vi "CRYSet Hardware Editor Front Panel.vi"(11 "Vi Ref":refnum<vi>) -> ()   [LabVIEW 2013]
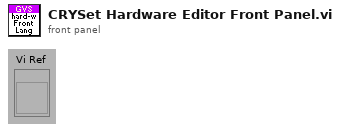
[diagram p1: front panel]
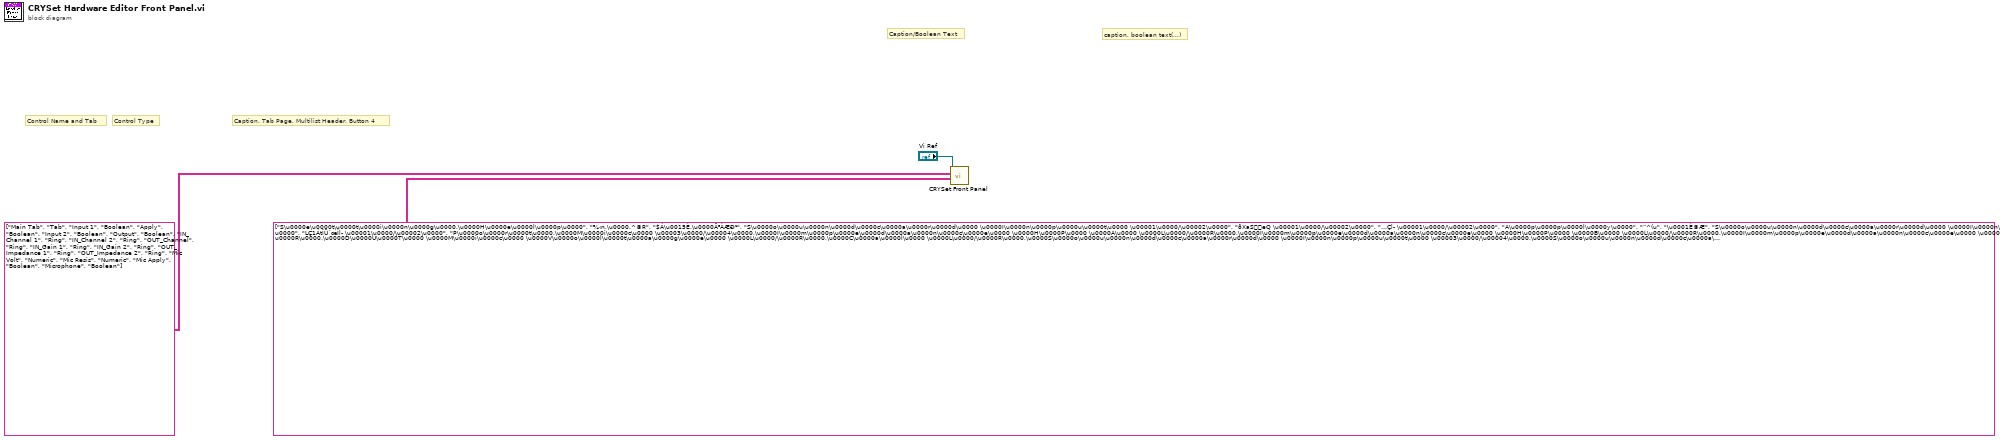
[diagram p0: block diagram]
diagram:
  # "Caption, Tab Page, Multilist Header, Button 4"
  # "Control Type"
  # "Control Name and Tab"
  # "caption, boolean text(,,,)"
  # "Caption/Boolean Text"
  n1 = call "CRYSet Front Panel.vi"("Caption(Boolean Text)"=string[][] [["S\u0000e\u0000t\u0000t\u0000i\u0000n\u0000g\u0000,\u0000H\u0000e\u0000l\u0000p\u0000", "¾‹n,\u0000.^©R", "$Á\u0015È,\u0000Ä³ÀÆÐ¹"], ["S\u0000o\u0000u\u0000n\u0000d\u0000c\u0000a\u0000r\u0000d\u0000 \u0000I\u0000n\u0000p\u0000u\u0000t\u0000 \u00001\u0000/\u00002\u0000", "ðXaSeQ \u00001\u0000/\u00002\u0000", "…Çl­ \u00001\u0000/\u00002\u0000"], ["A\u0000p\u0000p\u0000l\u0000y\u0000", "”^(u", "\u0001È©Æ"], ["S\u0000o\u0000u\u0000n\u0000d\u0000c\u0000a\u0000r\u0000d\u0000 \u0000I\u0000n\u0000p\u0000u\u0000t\u0000 \u00003\u0000/\u00004\u0000", "ðXaSeQ \u00003\u0000/\u00004\u0000", "LÇ1ÁtÎÜ´…Çl­ \u00001\u0000/\u00002\u0000"], ["S\u0000o\u0000u\u0000n\u0000d\u0000c\u0000a\u0000r\u0000d\u0000 \u0000O\u0000u\u0000t\u0000p\u0000u\u0000t\u0000 \u00001\u0000/\u00002\u0000", "ðXaSúQ \u00001\u0000/\u00002\u0000", "LÇ1ÁtÎÜ´œÍl­ \u00001\u0000/\u00002\u0000"], ["P\u0000o\u0000r\u0000t\u0000,\u0000M\u0000i\u0000c\u0000 \u00003\u0000/\u00004\u0000,\u0000I\u0000m\u0000p\u0000e\u0000d\u0000a\u0000n\u0000c\u0000e\u0000 \u0000H\u0000P\u0000 \u0000A\u0000 \u0000L\u0000/\u0000R\u0000,\u0000I\u0000m\u0000p\u0000e\u0000d\u0000a\u0000n\u0000c\u0000e\u0000 \u0000H\u0000P\u0000 \u0000B\u0000 \u0000L\u0000/\u0000R\u0000,\u0000I\u0000m\u0000p\u0000e\u0000d\u0000a\u0000n\u0000c\u0000e\u0000 \u0000H\u0000P\u0000 \u0000C\u0000 \u0000L\u0000/\u0000R\u0000,\u0000I\u0000m\u0000p\u0000e\u0000d\u0000a\u0000n\u0000c\u0000e\u0000 \u0000H\u0000P\u0000 \u0000D\u0000 \u0000L\u0000/\u0000R\u0000,\u0000D\u0000U\u0000T\u0000 \u0000M\u0000i\u0000c\u0000 \u0000C\u0000u\u0000r\u0000r\u0000e\u0000n\u0000t\u0000 \u0000L\u0000/\u0000R\u0000,\u0000D\u0000U\u0000T\u0000 \u0000M\u0000i\u0000c\u0000 \u0000V\u0000o\u0000l\u0000t\u0000a\u0000g\u0000e\u0000 \u0000L\u0000/\u0000R\u0000,\u0000C\u0000a\u0000l\u0000 \u0000L\u0000/\u0000R\u0000,\u0000S\u0000o\u0000u\u0000n\u0000d\u0000c\u0000a\u0000r\u0000d\u0000 \u0000I\u0000n\u0000p\u0000u\u0000t\u0000 \u00003\u0000/\u00004\u0000,\u0000S\u0000o\u0000u\u0000n\u0000d\u0000c\u0000a\u0000r\u0000d\u0000 \u0000O\u0000u\u0000t\u0000p\u0000u\u0000t\u0000 \u00001\u0000/\u00002\u0000,\u0000S\u0000o\u0000u\u0000n\u0000d\u0000c\u0000a\u0000r\u0000d\u0000 \u0000O\u0000u\u0000t\u0000p\u0000u\u0000t\u0000 \u00001\u0000(\u0000-\u00002\u00000\u0000d\u0000B\u0000)\u0000", "ïzãS,\u0000 OðXhV \u00003\u0000/\u00004\u0000,\u00003:g;b \u0000A\u0000 \u0000L\u0000/\u0000R\u0000,\u00003:g;b \u0000B\u0000 \u0000L\u0000/\u0000R\u0000,\u00003:g;b \u0000C\u0000 \u0000L\u0000/\u0000R\u0000,\u00003:g;b \u0000D\u0000 \u0000L\u0000/\u0000R\u0000,\u0000ªT4Y5uAm \u0000L\u0000/\u0000R\u0000,\u0000ªT4Y5uS \u0000L\u0000/\u0000R\u0000,\u0000Qè!hÆQáO÷S \u0000L\u0000/\u0000R\u0000,\u0000ðXaSeQ \u00003\u0000/\u00004\u0000,\u0000ðXaSúQ \u00001\u0000/\u00002\u0000,\u0000ðXaSúQ \u00001\u0000(\u0000-\u00002\u00000\u0000d\u0000B\u0000)\u0000", "ìÓ¸Ò,\u0000M\u0000i\u0000c\u0000 \u00003\u0000/\u00004\u0000,\u0000I\u0000m\u0000p\u0000 \u00001\u0000 \u0000L\u0000/\u0000R\u0000,\u0000I\u0000m\u0000p\u0000 \u00002\u0000 \u0000L\u0000/\u0000R\u0000,\u0000I\u0000m\u0000p\u0000 \u00003\u0000 \u0000L\u0000/\u0000R\u0000,\u0000I\u0000m\u0000p\u0000 \u00004\u0000 \u0000L\u0000/\u0000R\u0000,\u0000D\u0000U\u0000T\u0000 \u0000M\u0000i\u0000c\u0000 \u0000C\u0000u\u0000r\u0000r\u0000e\u0000n\u0000t\u0000 \u0000L\u0000/\u0000R\u0000,\u0000D\u0000U\u0000T\u0000 \u0000M\u0000i\u0000c\u0000 \u0000V\u0000o\u0000l\u0000t\u0000a\u0000g\u0000e\u0000 \u0000L\u0000/\u0000R\u0000,\u0000C\u0000a\u0000l\u0000 \u0000L\u0000/\u0000R\u0000,\u0000I\u0000n\u0000p\u0000u\u0000t\u0000 \u00003\u0000/\u00004\u0000,\u0000O\u0000u\u0000t\u0000p\u0000u\u0000t\u0000 \u00001\u0000/\u00002\u0000,\u0000O\u0000u\u0000t\u0000p\u0000u\u0000t\u0000 \u00001\u0000(\u0000-\u00002\u00000\u0000d\u0000B\u0000)\u0000"], ["P\u0000o\u0000r\u0000t\u0000,\u0000M\u0000i\u0000c\u0000 \u00001\u0000/\u00002\u0000,\u0000M\u0000i\u0000c\u0000 \u00003\u0000/\u00004\u0000,\u0000M\u0000i\u0000c\u0000 \u00005\u0000/\u00006\u0000,\u0000M\u0000i\u0000c\u0000 \u00007\u0000/\u00008\u0000,\u0000L\u0000i\u0000n\u0000e\u0000I\u0000n\u0000 \u0000L\u0000/\u0000R\u0000,\u0000D\u0000U\u0000T\u0000 \u0000M\u0000i\u0000c\u0000 \u0000L\u0000/\u0000R\u0000,\u0000I\u0000m\u0000p\u0000e\u0000d\u0000a\u0000n\u0000c\u0000e\u0000 \u0000H\u0000P\u0000 \u0000B\u0000 \u0000L\u0000/\u0000R\u0000,\u0000C\u0000a\u0000l\u0000 \u0000L\u0000/\u0000R\u0000", "ïzãS,\u0000 OðXhV \u00001\u0000/\u00002\u0000,\u0000 OðXhV \u00003\u0000/\u00004\u0000,\u0000 OðXhV \u00005\u0000/\u00006\u0000,\u0000 OðXhV \u00007\u0000/\u00008\u0000,\u0000¿~ïeQ \u0000L\u0000/\u0000R\u0000,\u0000ªT4Y \u0000L\u0000/\u0000R\u0000,\u00003:g;b \u0000B\u0000 \u0000L\u0000/\u0000R\u0000,\u0000Qè!hÆQáO÷S \u0000L\u0000/\u0000R\u0000", "ìÓ¸Ò,\u0000M\u0000i\u0000c\u0000 \u00001\u0000/\u00002\u0000,\u0000M\u0000i\u0000c\u0000 \u00003\u0000/\u00004\u0000,\u0000M\u0000i\u0000c\u0000 \u00005\u0000/\u00006\u0000,\u0000M\u0000i\u0000c\u0000 \u00007\u0000/\u00008\u0000,\u0000L\u0000i\u0000n\u0000e\u0000I\u0000n\u0000 \u0000L\u0000/\u0000R\u0000,\u0000D\u0000U\u0000T\u0000 \u0000M\u0000i\u0000c\u0000 \u0000L\u0000/\u0000R\u0000,\u0000I\u0000m\u0000p\u0000 \u00002\u0000 \u0000L\u0000/\u0000R\u0000,\u0000C\u0000a\u0000l\u0000 \u0000L\u0000/\u0000R\u0000"], ["P\u0000o\u0000r\u0000t\u0000,\u0000M\u0000o\u0000u\u0000t\u0000h\u0000 \u0000S\u0000i\u0000m\u0000u\u0000l\u0000a\u0000t\u0000o\u0000r\u0000 \u00001\u0000,\u0000M\u0000o\u0000u\u0000t\u0000h\u0000 \u0000S\u0000i\u0000m\u0000u\u0000l\u0000a\u0000t\u0000o\u0000r\u0000 \u00002\u0000,\u0000H\u0000e\u0000a\u0000d\u0000p\u0000h\u0000o\u0000n\u0000e\u0000 \u0000A\u0000/\u0000B\u0000,\u0000H\u0000e\u0000a\u0000d\u0000p\u0000h\u0000o\u0000n\u0000e\u0000 \u0000A\u0000/\u0000B\u0000(\u0000L\u0000=\u0000R\u0000)\u0000", "ïzãS,\u0000ÿN\u001fw4V \u00001\u0000,\u0000ÿN\u001fw4V \u00002\u0000,\u00003€:g \u0000A\u0000/\u0000B\u0000,\u00003€:g \u0000A\u0000/\u0000B\u0000(\u0000L\u0000=\u0000R\u0000)\u0000", "ìÓ¸Ò"], ["G\u0000a\u0000i\u0000n\u0000", ">e'Y", "ÉíÓ"], ["G\u0000a\u0000i\u0000n\u0000", ">e'Y", "ÉíÓ"], ["I\u0000m\u0000p\u0000e\u0000d\u0000a\u0000n\u0000c\u0000e\u0000 \u0000H\u0000P\u0000 \u0000A\u0000,\u00001\u0000,\u00003\u00003\u0000 \u0000D\u0000i\u0000f\u0000f\u0000e\u0000r\u0000e\u0000n\u0000t\u0000i\u0000a\u0000l\u0000,\u00003\u00003\u0000 \u0000S\u0000i\u0000n\u0000g\u0000l\u0000e\u0000-\u0000E\u0000n\u0000d\u0000,\u00001\u00005\u00000\u0000,\u00006\u00000\u00000\u0000,\u00007\u00005\u00000\u0000", "3€:g;–—b \u0000A\u0000,\u00001\u0000,\u00003\u00003\u0000 \u0000î]\u0006R,\u00003\u00003\u0000 \u0000USïz,\u00001\u00005\u00000\u0000,\u00006\u00000\u00000\u0000,\u00007\u00005\u00000\u0000", "3€:g;–—b \u0000A\u0000,\u00001\u0000,\u00003\u00003\u0000 \u0000î]\u0006R,\u00003\u00003\u0000 \u0000USïz,\u00001\u00005\u00000\u0000,\u00006\u00000\u00000\u0000,\u00007\u00005\u00000\u0000"], ["I\u0000m\u0000p\u0000e\u0000d\u0000a\u0000n\u0000c\u0000e\u0000 \u0000H\u0000P\u0000 \u0000B\u0000", "3€:g;–—b \u0000B\u0000", "\u0000ÈmÕ \u00002\u0000"], ["M\u0000i\u0000c\u0000 \u0000V\u0000o\u0000l\u0000t\u0000", "ªT4Y5u‹S", "È¹tÇlÐ\u0004ÈUÅ"], ["M\u0000i\u0000c\u0000 \u0000R\u0000e\u0000s\u0000i\u0000s\u0000", "ªT4Y5u;–", "È¹tÇlÐ\u0000ÈmÕ"], ["M\u0000i\u0000c\u0000 \u0000A\u0000p\u0000p\u0000l\u0000y\u0000", "ªT4Y5u;–5u‹Snxš[", "È¹tÇlÐ\u0001È©Æ"], ["M\u0000i\u0000c\u0000r\u0000o\u0000p\u0000h\u0000o\u0000n\u0000e\u0000", "ªT4Y", "È¹tÇlÐ\\¸ðÓ"]], "Control ID and Type(Label Name, Type)"=string[][] [["Main Tab", "Tab"], ["Input 1", "Boolean"], ["Apply", "Boolean"], ["Input 2", "Boolean"], ["Output", "Boolean"], ["IN_Channel 1", "Ring"], ["IN_Channel 2", "Ring"], ["OUT_Channel", "Ring"], ["IN_Gain 1", "Ring"], ["IN_Gain 2", "Ring"], ["OUT_Impedance 1", "Ring"], ["OUT_Impedance 2", "Ring"], ["Mic Volt", "Numeric"], ["Mic Resis", "Numeric"], ["Mic Apply", "Boolean"], ["Microphone", "Boolean"]], "Vi Ref"="Vi Ref") -> ()  [unwired: 9 in]
